vi "MGCC_FntStaMach_Flagtoevent_PhaseTwo.vi"(0 "Island_status":bool, 1 "M_OFF":bool, 2 "ABN_state":string, 3 "ABN_recover":bool, 5 "planned_isd":bool, 7 "Flags":bool[](array[boolean]), 9 "Pre_state":string, 11 "BKS_s":bool, 12 "UnplanBKS":bool, 13 "ISD_success":bool, 14 "Check_time":bool) -> (6 "Previous_state":string, 8 "error out":errorcluster, 10 "Event":bool[](array[boolean]))   [LabVIEW 2016]
uses:
  <vilib>/imath/engines/lvmath/Plug In/_Char/NIMS_CH_character datatype.ctl
  <vilib>/imath/engines/lvmath/Plug In/_Char/NIMS_CH_String to Character Array.vi
  <vilib>/imath/engines/lvmath2/RunTimeEngine/IndexRead/NIMS V(S).vi
  <instcachedir>/0/NIMS V(S)_0488751826AF41519A22953C041130DC.lvgen/NIMS V(S)_0488751826AF41519A22953C041130DC_003.vi
  <vilib>/imathl/engines/lvmath/Functions/Error Handling/Create Error.vi
  <vilib>/imath/engines/lvmath2/RunTimeSupport/NIMS_Compare Aggregates.vi
  <instcachedir>/0/NIMS_Compare Aggregates_FA3EBEB3749E48D38A57888B5ABBF163.lvgen/NIMS_Compare Aggregates_FA3EBEB3749E48D38A57888B5ABBF163_000.vi
  <vilib>/imath/engines/lvmath2/RunTimeEngine/NodeEndStatement/NIMS_NodeEndStatement_Output.vi
  <instcachedir>/0/NIMS_NodeEndStatement_Output_53EC0D466D134D7ABD903AC30B43404B.lvgen/NIMS_NodeEndStatement_Output_53EC0D466D134D7ABD903AC30B43404B_013.vi
  <vilib>/imath/engines/lvmath/Plug In/_Char/NIMS_CH_Character RV to String.vi
  <instcachedir>/0/NIMS_NodeEndStatement_Output_53EC0D466D134D7ABD903AC30B43404B.lvgen/NIMS_NodeEndStatement_Output_53EC0D466D134D7ABD903AC30B43404B_008.vi
  <vilib>/imath/engines/lvmath2/RunTimeEngine/ErrorHandling/NIMS_Finalize Error.vi
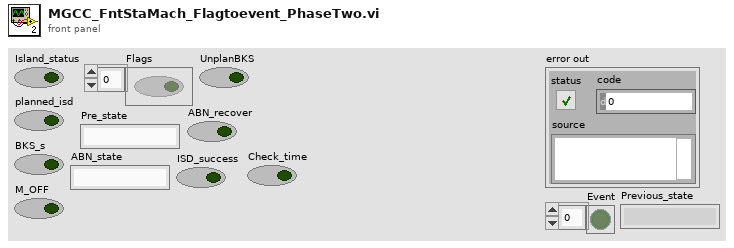
[diagram p1: front panel]
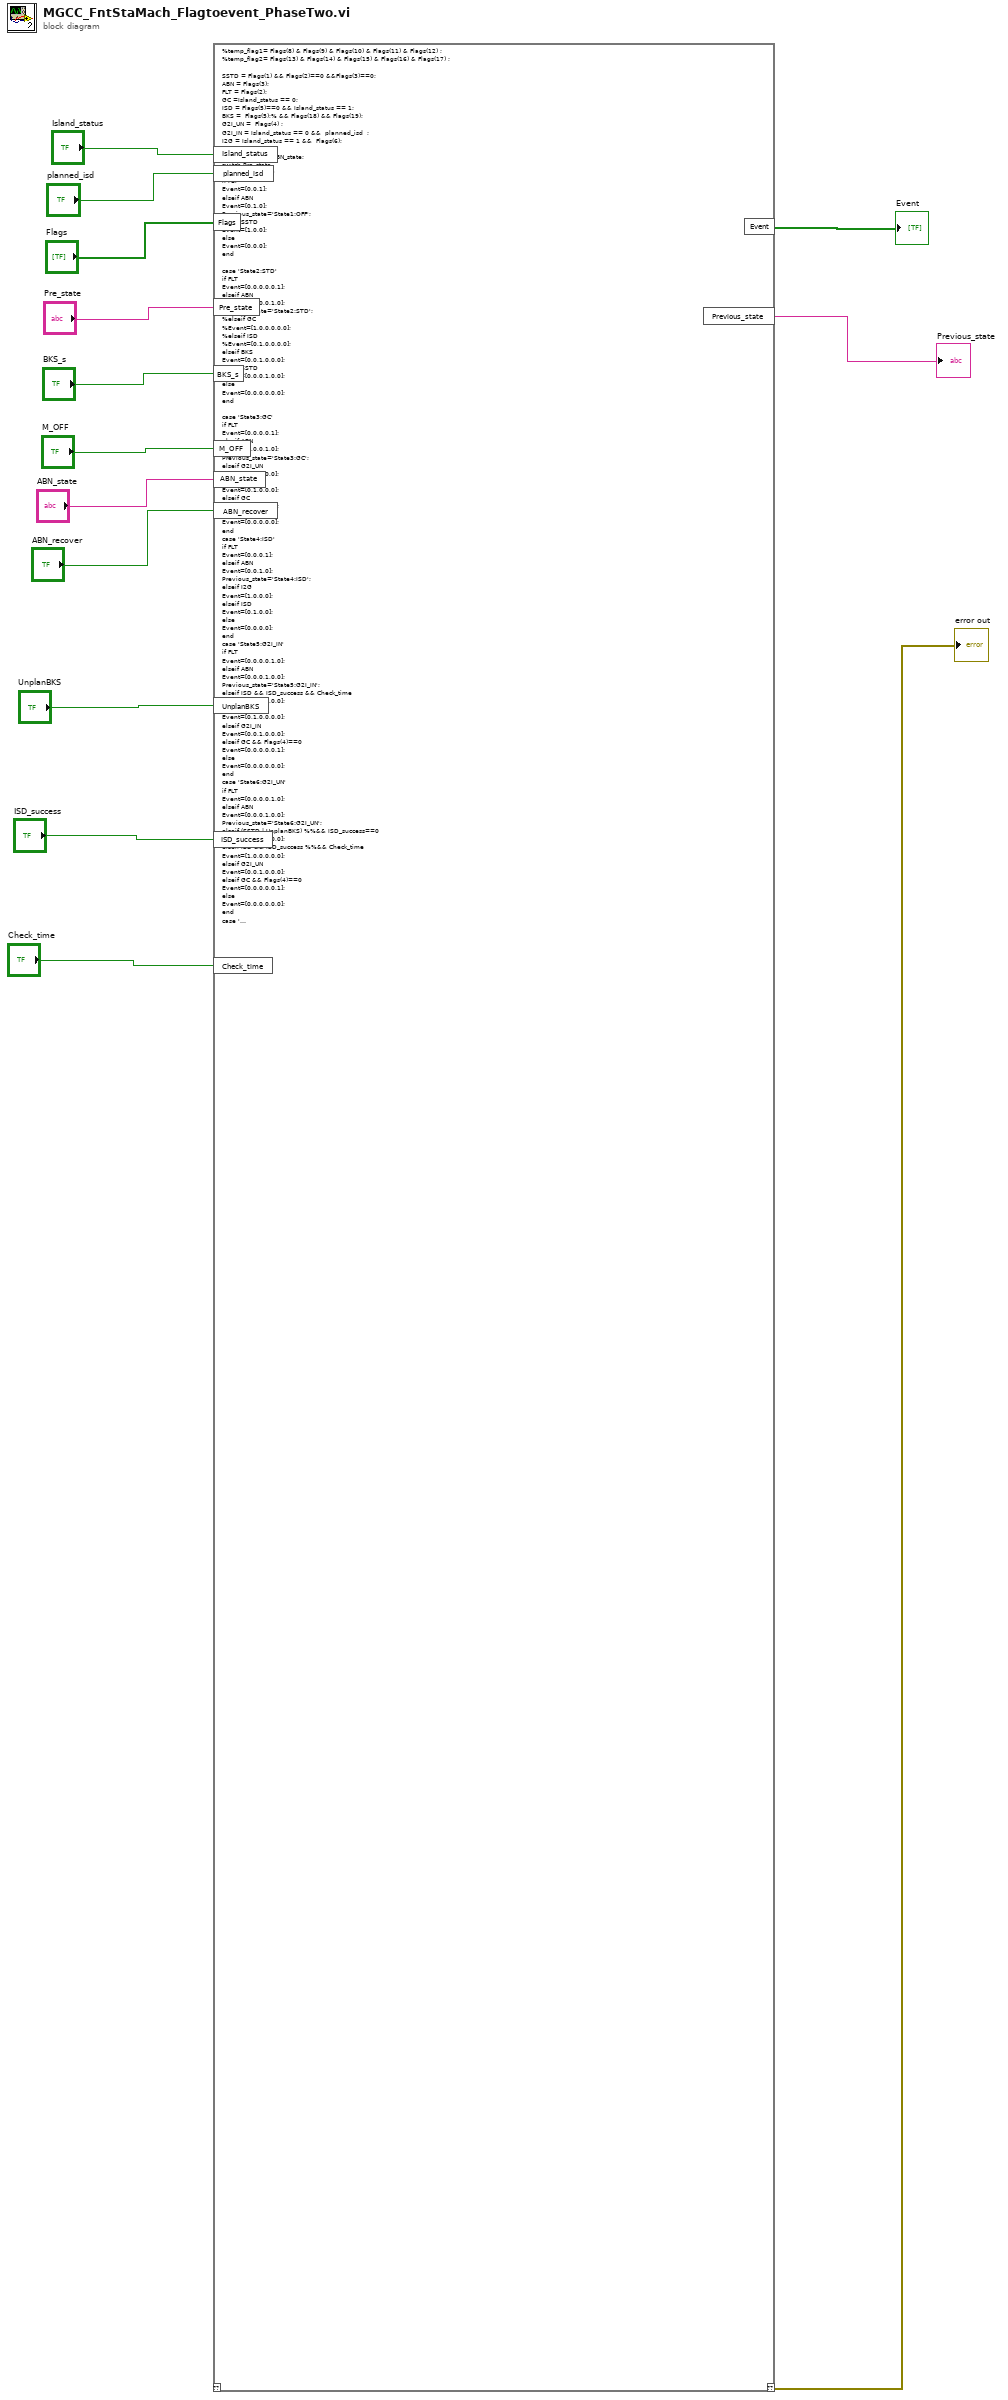
[diagram p0: block diagram]
diagram:
  n1 = mathscript code="%temp_flag1= Flags(8) & Flags(9) & Flags(10) & Flags(11) & Flags(12) ;\n%temp_flag2= Flags(13) & Flags(14) & Flags(15) & Flags(16) & Flags(17) ;\n\nSSTD = Flags(1) && Flags(2)==0 &&Flags(3)==0;\nABN = Flags(3);\nFLT = Flags(2);\nGC =Island_status == 0;\nISD = Flags(5)==0 && Island_status == 1;\nBKS =  Flags(5);% && Flags(18) && Flags(19);\nG2I_UN =  Flags(4) ;\nG2I_IN = Island_status == 0 &&  planned_isd  ;\nI2G = Island_status == 1 &&  Flags(6);\nOFF = M_OFF;\nPrevious_state=ABN_state;\nswitch Pre_state\ncase 'State1:OFF'\nif FLT\nEvent=[0,0,1];\nelseif ABN\nEvent=[0,1,0];\nPrevious_state='State1:OFF';\nelseif SSTD\nEvent=[1,0,0];\nelse\nEvent=[0,0,0];\nend \n\ncase 'State2:STD'\nif FLT\nEvent=[0,0,0,0,0,1];\nelseif ABN\nEvent=[0,0,0,0,1,0];\nPrevious_state='State2:STD';\n%elseif GC\n%Event=[1,0,0,0,0,0];\n%elseif ISD\n%Event=[0,1,0,0,0,0];\nelseif BKS\nEvent=[0,0,1,0,0,0];\nelseif SSTD\nEvent=[0,0,0,1,0,0];\nelse\nEvent=[0,0,0,0,0,0];\nend \n\ncase 'State3:GC'\nif FLT\nEvent=[0,0,0,0,1];\nelseif ABN\nEvent=[0,0,0,1,0];\nPrevious_state='State3:GC';\nelseif G2I_UN\nEvent=[1,0,0,0,0];\nelseif G2I_IN\nEvent=[0,1,0,0,0];\nelseif GC\nEvent=[0,0,1,0,0];\nelse\nEvent=[0,0,0,0,0];\nend\ncase 'State4:ISD'\nif FLT\nEvent=[0,0,0,1];\nelseif ABN\nEvent=[0,0,1,0];\nPrevious_state='State4:ISD';\nelseif I2G\nEvent=[1,0,0,0];\nelseif ISD\nEvent=[0,1,0,0];\nelse\nEvent=[0,0,0,0];\nend\ncase 'State5:G2I_IN'\nif FLT\nEvent=[0,0,0,0,1,0];\nelseif ABN\nEvent=[0,0,0,1,0,0];\nPrevious_state='State5:G2I_IN';\nelseif ISD && ISD_success && Check_time\nEvent=[1,0,0,0,0,0];\nelseif SSTD\nEvent=[0,1,0,0,0,0];\nelseif G2I_IN\nEvent=[0,0,1,0,0,0];\nelseif GC && Flags(4)==0 \nEvent=[0,0,0,0,0,1];\nelse\nEvent=[0,0,0,0,0,0];\nend\ncase 'State6:G2I_UN'\nif FLT\nEvent=[0,0,0,0,1,0];\nelseif ABN\nEvent=[0,0,0,1,0,0];\nPrevious_state='State6:G2I_UN';\nelseif (SSTD | UnplanBKS) %%&& ISD_success==0\nEvent=[0,1,0,0,0,0];\nelseif ISD && ISD_success %%&& Check_time\nEvent=[1,0,0,0,0,0];\nelseif G2I_UN\nEvent=[0,0,1,0,0,0];\nelseif GC && Flags(4)==0 \nEvent=[0,0,0,0,0,1];\nelse\nEvent=[0,0,0,0,0,0];\nend\ncase 'State7:I2G'\nif FLT\nEvent=[0,0,0,0,1,0];\nelseif ABN\nEvent=[0,0,0,1,0,0];\nPrevious_state='State7:I2G';\nelseif GC\nEvent=[1,0,0,0,0,0];\nelseif SSTD\nEvent=[0,1,0,0,0,0];\nelseif I2G\nEvent=[0,0,1,0,0,0];\nelseif ISD && Flags(6) ==0\nEvent=[0,0,0,0,0,1];\nelse\nEvent=[0,0,0,0,0,0];\nend\ncase 'State8:BKS'\nif FLT\nEvent=[0,0,0,0,1];\nelseif ABN\nEvent=[0,0,0,1,0];\nPrevious_state='State8:BKS';\nelseif ISD && BKS_s\nEvent=[1,0,0,0,0];\nelseif SSTD\nEvent=[0,1,0,0,0];\nelseif BKS\nEvent=[0,0,1,0,0];\nelse\nEvent=[0,0,0,0,0];\nend\ncase 'State9:ABN'\nif FLT\nEvent=[0,0,0,0,0,0,0,0,1];\nelseif ABN\nEvent=[0,0,0,0,0,0,0,1,0];\nelse\nswitch ABN_state\ncase 'State2:STD'\nEvent=[1,0,0,0,0,0,0,0,0];\ncase 'State3:GC'\nEvent=[0,1,0,0,0,0,0,0,0];\ncase 'State4:ISD'\nEvent=[0,0,1,0,0,0,0,0,0];\ncase 'State6:G2I_UN'\nEvent=[0,0,0,0,1,0,0,0,0];\ncase 'State5:G2I_IN'\nEvent=[0,0,0,1,0,0,0,0,0];\ncase 'State7:I2G'\nEvent=[0,0,0,0,0,1,0,0,0];\ncase 'State8:BKS'\nEvent=[0,0,0,0,0,0,1,0,0];\notherwise\nEvent=[0,0,0,0,0,0,0,1,0];\nend\nend\n\ncase 'State10:FLT'\nif FLT\nEvent=[1,0,0,0];\nelseif ABN\nEvent=[0,1,0,0];\nelseif SSTD\nEvent=[0,0,1,0];\nelseif OFF\nEvent=[0,0,0,1];\nelse\nEvent=[0,0,0,0];\nend\notherwise\nEvent=[0,0,0,0,0,0,0,1,0];\nend"("Flags"="Flags", "Pre_state"="Pre_state", "M_OFF"="M_OFF", "BKS_s"="BKS_s", "Island_status"="Island_status", "ABN_state"="ABN_state", "ABN_recover"="ABN_recover", "planned_isd"="planned_isd", "UnplanBKS"="UnplanBKS", "ISD_success"="ISD_success", "Check_time"="Check_time") -> ("??"=→"error out":errorcluster, "Event"=→"Event":bool[], "Previous_state"=→"Previous_state":string)  [unwired: 1 in]
